vi "Configuration parameter writing.vi"(7 "运行模式":enum16{"维护模式", "常规模式"}(ring)=enum."常规模式", 8 "error in (no error)":errorcluster caption="错误输入（无错误）", 9 "串口打开":bool, 10 "baud rate (9600)":u32(ring)=19200 caption="波特率" items=["1200"=1200, "2400"=2400, "4800"=4800, "9600"=9600, "19200"=19200, "38400"=38400, "115200"=115200], 11 "VISA resource name":refnum<visa-resource-name> caption="串口") -> (0 "error out":errorcluster caption="错误输出")   [LabVIEW 2016, in "SL1500-3G.lvlib"]
uses:
  SL1500-3G.lvlib
  <vilib>/Utility/config.llb/Write Key (I32).vi
  <vilib>/Utility/config.llb/Write Key (Boolean).vi
  <vilib>/Utility/config.llb/Write Key (String).vi
  <vilib>/Utility/config.llb/Write Key (U32).vi
  <vilib>/Utility/config.llb/NI_LVConfig.lvlib
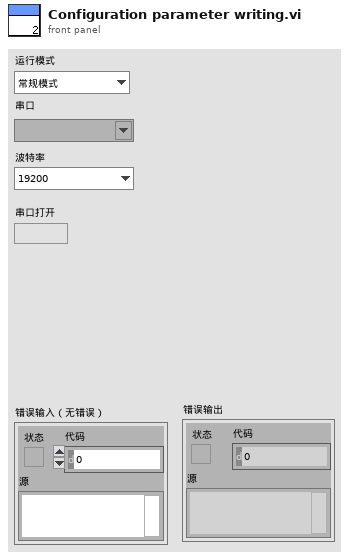
[diagram p1: front panel]
types:
  T1 = typedef "NI_LVConfig.lvlib/Config Data RefNum.ctl" = refnum<k1>
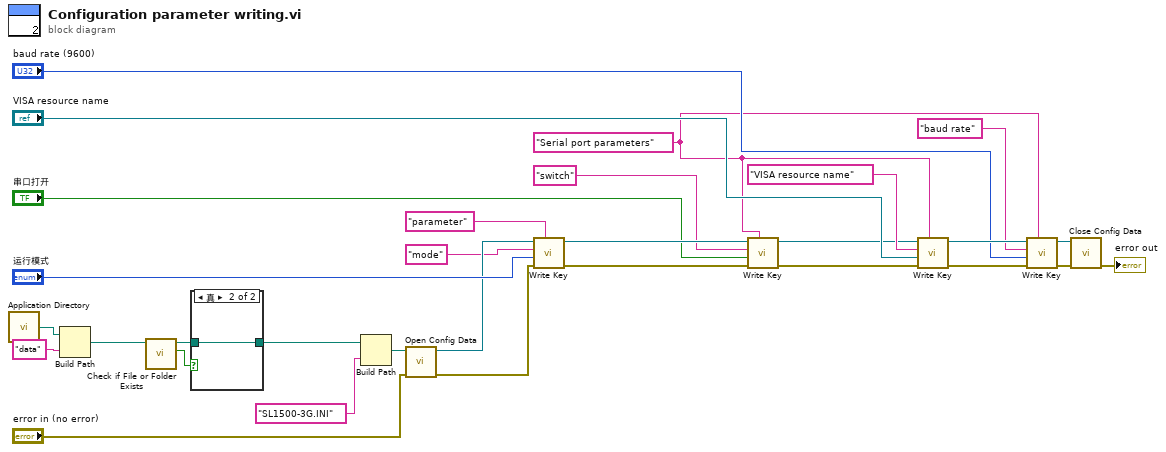
[diagram p0: block diagram]
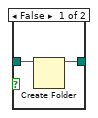
[diagram p2: hidden frame]
diagram:
  w5 = "Serial port parameters" ("section")
  n1 = call <vilib>:"Application Directory.vi"() -> ("Application Directory"=w18:path)
  n2 = Build Path(base path=w18, name or relative path="data" ("名称或相对路径")) -> (appended path=w16:path)
  n3 = call <vilib>:"Check if File or Folder Exists.vi"("path"=w16) -> ("file or folder exists?"=w15:bool, "dup path"=w14:path)  [unwired: 8 in, 1 out]
  n4 = case shown="真" w15 {
    tunnel: w14 -> [w32 w33]
    tunnel: [w31 w33] -> w13
    frame False {
      n5 = Create Folder(path (use dialog)=w32) -> (created path=w31:path)  [unwired: 2 in, 2 out]
    }
    frame True {
    }
  }
  n6 = Build Path(base path=w13, name or relative path="SL1500-3G.INI" ("名称或相对路径")) -> (appended path=w30:path)
  n7 = call <vilib>:"Open Config Data.vi"("error in (no error)"="error in (no error)", "configuration file path"=w30) -> ("error out"=w9:errorcluster, "refnum"=w7:T1)  [unwired: 7 in, 1 out]
  n8 = call-poly <vilib>:"Write Key.vi"("section"="parameter", "error in (no error)"=w9, "value"="运行模式", "key"="mode", "refnum"=w7) -> ("error out"=w11:errorcluster, "refnum out"=w12:T1)  [unwired: 4 in, 1 out]
  n9 = call-poly <vilib>:"Write Key.vi"("section"=w5, "error in (no error)"=w11, "value"="串口打开", "key"="switch", "refnum"=w12) -> ("error out"=w8:errorcluster, "refnum out"=w6:T1)  [unwired: 4 in, 1 out]
  n10 = call-poly <vilib>:"Write Key.vi"("section"=w5, "error in (no error)"=w8, "value"="VISA resource name", "key"="VISA resource name", "refnum"=w6) -> ("error out"=w26:errorcluster, "refnum out"=w27:T1)  [unwired: 4 in, 1 out]
  n11 = call-poly <vilib>:"Write Key.vi"("section"=w5, "error in (no error)"=w26, "value"="baud rate (9600)", "key"="baud rate", "refnum"=w27) -> ("error out"=w23:errorcluster, "refnum out"=w24:T1)  [unwired: 4 in, 1 out]
  n12 = call <vilib>:"Close Config Data.vi"("error in (no error)"=w23, "refnum"=w24) -> ("error out"=→"error out":errorcluster)  [unwired: 8 in, 1 out]
